vi "testHardpoint.vi"(8 "error in (no error)":errorcluster, 9 "Parameters":T1, 10 "Model in":refnum<class "Model.lvclass">, 11 "State in":refnum<class "State.lvclass">) -> (0 "error out":errorcluster, 2 "Model out":refnum<class "Model.lvclass">, 3 "State out":refnum<class "State.lvclass">)   [LabVIEW 2016, in "State.lvclass"]
uses:
  State.lvclass
  Model/Model.lvclass
  DataTypes/Topics/CommandTestHardpoint.ctl
  DataTypes/Topics/Parts/CommandId.ctl
  DataTypes/Topics/M1M3SupportTopics.lvlib
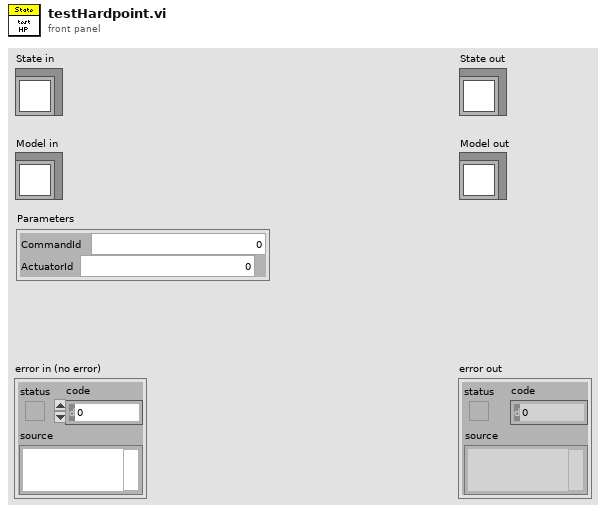
[diagram p1: front panel]
types:
  T1 = typedef "M1M3SupportTopics.lvlib/CommandTestHardpoint.ctl" = cluster{"CommandId":T2, "ActuatorId":i32}
  T2 = typedef "M1M3SupportTopics.lvlib/CommandId.ctl" = i32
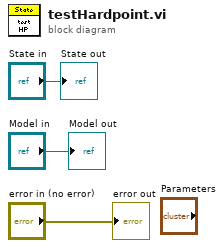
[diagram p0: block diagram]
diagram:
  "error out" <- "error in (no error)"
  "State out" <- "State in"
  "Model out" <- "Model in"
